vi "Initialize.vi"(7 "Configure RS232 Baud Rate":u32(ring)=115200 items=["9600"=9600, "19200"=19200, "38400"=38400, "57600"=57600, "115200"=115200], 8 "error in (no error)":errorcluster, 9 "Clear Error(True)":bool=TRUE, 10 "ID Query (True)":bool=TRUE, 11 "VISA resource name":refnum<visa-resource-name>) -> (0 "error out":errorcluster, 1 "ID Return Count":i32, 2 "ID Return String":string, 3 "VISA resource name out":refnum<visa-resource-name>)   [LabVIEW 2021, in "DMM4.lvlib"]
doc: "Establishes communication with the instrument and optionally performs an instrument identification query and/or an instrument reset. It also places the instrument in a default state needed for other instrument driver operations. Therefore, call this VI before calling other instrument driver VIs for this instrument. Generally, you need to call the Initialize VI only once at the beginning of an application."
uses:
  DMM4.lvlib
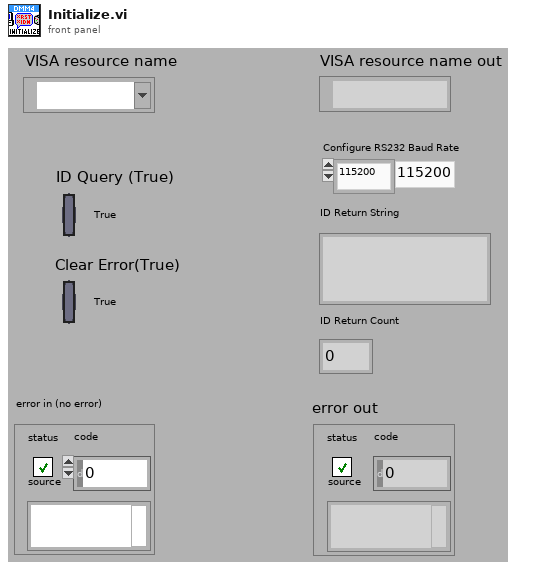
[diagram p1: front panel]
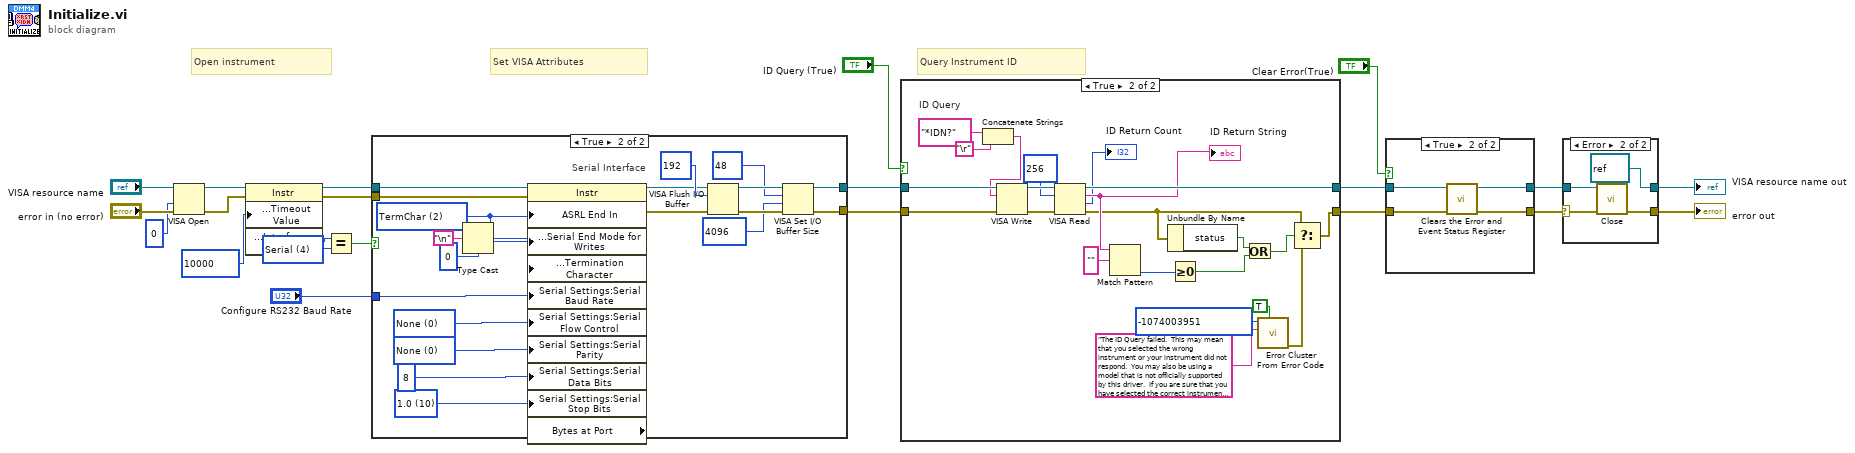
[diagram p0: block diagram]
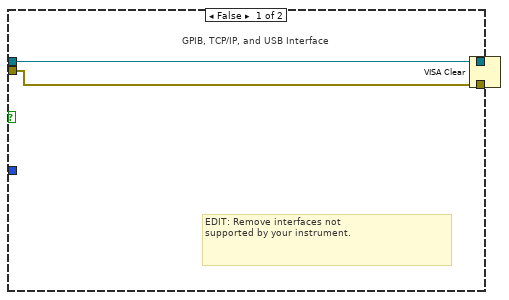
[diagram p2: hidden frame]
diagram:
  w12 = u16 4 items=["GPIB"=1, "VXI"=2, "GPIB-VXI"=3, "Serial"=4, "PXI"=5, "TCPIP"=6, "USB"=7] ("Interface Information:Interface Type")
  # "Set VISA Attributes"
  # "Query Instrument ID"
  # "Open instrument"
  n1 = VISA Open(access mode=u32 0, error in (no error)="error in (no error)", VISA resource name="VISA resource name") -> (VISA resource name=w2:refnum<visa-resource-name>, error out=w1:errorcluster)  [unwired: 2 in]
  n2 = property class="Instr"(reference=w2, error in=w1, "General Settings:Timeout Value"=u32 10000) -> (reference out=w15:refnum<visa-resource-name>, error out=w14:errorcluster, "Interface Information:Interface Type"=w18:u16)
  n3 = Equal?(x=w18, y=w12) -> (x = y?=w13:bool)
  n4 = case shown="True" w13 {
    tunnel: [w25 w28] -> w16
    tunnel: [w23 w27] -> w6
    tunnel: w15 -> [w26 w45]
    tunnel: w14 -> [w24 w46]
    tunnel: "Configure RS232 Baud Rate" -> [_ w32]
    frame False {
      # "EDIT: Remove interfaces not\nsupported by your instrument."
      # "GPIB, TCP/IP, and USB Interface"
      n5 = VISA Clear(VISA resource name=w26, error in (no error)=w24) -> (VISA resource name out=w25:refnum<visa-resource-name>, error out=w23:errorcluster)
    }
    frame True {
      w35 = u16 10 items=["1.0"=10, "1.5"=15, "2.0"=20] ("Serial Settings:Stop Bits")
      w33 = u16 0 items=["None", "Odd", "Even", "Mark", "Space"] ("Serial Settings:Parity")
      w34 = u16 0 items=["None", "XON/XOFF", "RTS/CTS", "XON/XOFF & RTS/CTS", "DTR/DSR", "XON/XOFF & DTR/DSR"] ("Serial Settings:Flow Control")
      w31 = u16 2 items=["None", "LastBit", "TermChar"] ("Serial Settings:Serial End Mode for Reads")
      # "Serial Interface"
      n6 = Type Cast(type=u8 0, x="\n") -> (*(type *) &x=w37:u8)
      n7 = property class="Instr" props=["ASRL End In", "Serial Settings:Serial End Mode for Writes", "Message Based Settings:Termination Character", "Serial Settings:Serial Baud Rate", "Serial Settings:Serial Flow Control", "Serial Settings:Serial Parity", "Serial Settings:Serial Data Bits", "Serial Settings:Serial Stop Bits", "Bytes at Port"](reference=w45, error in=w46, "ASRL End In"=w31, "Serial Settings:Serial End Mode for Writes"=w31, "Message Based Settings:Termination Character"=w37, "Serial Settings:Serial Baud Rate"=w32, "Serial Settings:Serial Flow Control"=w34, "Serial Settings:Serial Parity"=w33, "Serial Settings:Serial Data Bits"=u16 8 ("Serial Settings:Data Bits"), "Serial Settings:Serial Stop Bits"=w35) -> (reference out=w30:refnum<visa-resource-name>, error out=w29:errorcluster)  [unwired: 1 out]
      n8 = VISA Flush I/O Buffer(VISA resource name=w30, mask (16)=u16 192, error in (no error)=w29) -> (VISA resource name out=w44:refnum<visa-resource-name>, error out=w43:errorcluster)
      n9 = VISA Set I/O Buffer Size(VISA resource name=w44, mask (16)=u16 48, size (4096)=u32 4096 ("size (0)"), error in (no error)=w43) -> (VISA resource name out=w28:refnum<visa-resource-name>, error out=w27:errorcluster)
    }
  }
  n10 = case shown="True" "ID Query (True)" {
    tunnel: [w47 w70] -> w21
    tunnel: [w48 w67] -> w22
    tunnel: w16 -> [w48 w68]
    tunnel: w6 -> [w47 w69]
    frame False {
    }
    frame True {
      w51 = "*IDN?"  # ID Query
      n11 = Concatenate Strings(w51, "\r" ("string")) -> (w49:string)
      n12 = VISA Write(VISA resource name=w68, write buffer=w49, error in (no error)=w69) -> (VISA resource name out=w66:refnum<visa-resource-name>, error out=w65:errorcluster)  [unwired: 1 out]
      n13 = VISA Read(VISA resource name=w66, byte count=u32 256, error in (no error)=w65) -> (VISA resource name out=w67:refnum<visa-resource-name>, read buffer=w54:string, return count=→"ID Return Count":u32, error out=w52:errorcluster)
      "ID Return String" <- w54
      n14 = Match Pattern(string=w54, regular expression="") -> (offset past match=w58:i32)  [unwired: 1 in, 3 out]
      n15 = Unbundle By Name(w52) -> ("status"=w57:bool)
      n16 = Greater Or Equal To 0?(x=w58) -> (x >= 0?=w56:bool)
      n17 = Or(x=w57, y=w56) -> (x .or. y?=w55:bool)
      n18 = call <vilib>:"Error Cluster From Error Code.vi"("show call chain? (False)"=TRUE, "error message (\"\")"="The ID Query failed.  This may mean that you selected the wrong instrument or your instrument did not respond.  You may also be using a model that is not officially supported by this driver.  If you are sure that you have selected the correct instrument and it is responding, try disabling the ID Query." ("Source (VI Name)"), "error code (0)"=-1074003951 ("Code")) -> ("error out"=w62:errorcluster)  [unwired: 6 in]
      n19 = Select(t=w52, s=w55, f=w62) -> (s? t:f=w70:errorcluster)
    }
  }
  n20 = case shown="True" "Clear Error(True)" {
    tunnel: w21 -> [w71 w76]
    tunnel: [w71 w73] -> w8
    tunnel: w22 -> [w72 w75]
    tunnel: [w72 w74] -> w9
    frame False {
    }
    frame True {
      n21 = call "Clears the Error and Event Status Register.vi"("error in (no error)"=w76, "VISA resource name"=w75) -> ("error out"=w73:errorcluster, "VISA resource name out"=w74:refnum<visa-resource-name>)  [unwired: 8 in]
    }
  }
  n22 = case shown="Error" w8 {
    selector: w8 -> [w77 w80]
    tunnel: w9 -> [w78 w81]
    tunnel: [w78 refnum<visa-resource-name> refnum ("VISA resource name out")] -> w11
    tunnel: [w77 w82] -> w10
    frame No Error {
    }
    frame Error {
      n23 = call "Close.vi"("error in (no error)"=w80, "VISA resource name"=w81) -> ("error out"=w82:errorcluster)  [unwired: 9 in]
    }
  }
  "VISA resource name out" <- w11
  "error out" <- w10
